vi "initialization.vi"(9 "软件版本":refnum<vi>, 10 "updateconfiguration":refnum<vi>) -> ()   [LabVIEW 2016, in "数据传输系统-02.lvlib"]
uses:
  <vilib>/Utility/config.llb/Read Key (String).vi
  <vilib>/Utility/config.llb/NI_LVConfig.lvlib
  update/update.lvlib
panel:
  in  "参数数值":T1={"CODMn"=TRUE, "CODCr"=TRUE, "DO"=TRUE, "铜"=TRUE, "PH"=TRUE, "氨氮"=TRUE, "比电导率"=TRUE, "水温"=TRUE, "COD"=TRUE, "浊度"=TRUE, "总氮"=TRUE, "总磷"=TRUE, "叶绿素a"=TRUE, "藻密度"=TRUE, "水位"=TRUE, "流速"=TRUE, "瞬时流量"=TRUE, "累积流量"=TRUE, "亚硝氮"=TRUE, "硫化物"=TRUE, "ORP"=TRUE, "铅"=TRUE, "镉"=TRUE, "锌"=TRUE, "镍"=TRUE, "锰"=TRUE, "汞"=TRUE, "气温"=TRUE, "气压"=TRUE, "风速"=TRUE, "风向"=TRUE, "盐度"=TRUE, "磷酸盐"=TRUE, "硝氮"=TRUE, "氟化物"=TRUE}
  out "配置表格":string[][](table)
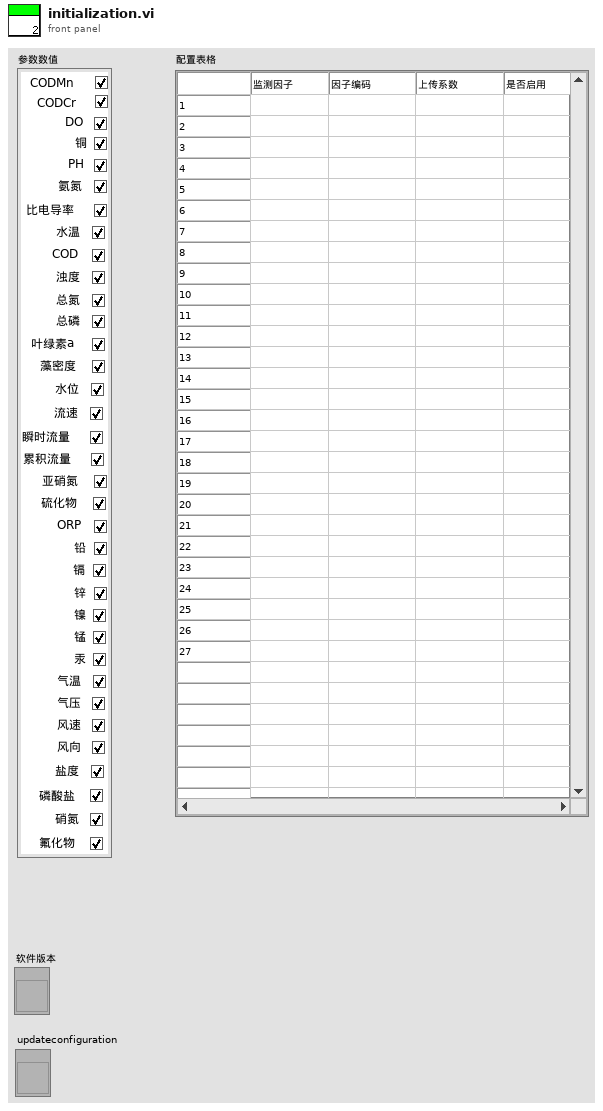
[diagram p1: front panel]
types:
  T1 = cluster{"CODMn":bool, "CODCr":bool, "DO":bool, "铜":bool, "PH":bool, "氨氮":bool, "比电导率":bool, "水温":bool, "COD":bool, "浊度":bool, "总氮":bool, "总磷":bool, "叶绿素a":bool, "藻密度":bool, "水位":bool, "流速":bool, "瞬时流量":bool, "累积流量":bool, "亚硝氮":bool, "硫化物":bool, "ORP":bool, "铅":bool, "镉":bool, "锌":bool, "镍":bool, "锰":bool, "汞":bool, "气温":bool, "气压":bool, "风速":bool, "风向":bool, "盐度":bool, "磷酸盐":bool, "硝氮":bool, "氟化物":bool}
  T2 = cluster{"setini":string, "sysini":string, "hechaini":string, "actualwrite":string, "actualread":string, "datasent":string, "反控命令信息队列":string, "反控与仪器交互":string}
  T3 = cluster{"CODMn":string, "CODCr":string, "DO":string, "铜":string, "PH":string, "氨氮":string, "比电导率":string, "水温":string, "COD":string, "浊度":string, "总氮":string, "总磷":string, "叶绿素a":string, "藻密度":string, "水位":string, "流速":string, "瞬时流量":string, "累积流量":string, "亚硝酸盐":string, "硫化物":string, "ORP":string, "铅":string, "镉":string, "锌":string, "镍":string, "锰":string, "汞":string, "气温":string, "气压":string, "风速":string, "风向":string, "盐度":string, "磷酸盐":string, "硝氮":string, "氟化物":string}
  T4 = typedef "NI_LVConfig.lvlib/Config Data RefNum.ctl" = refnum<k1>
  T5 = cluster{"[0]":string, "[1]":string, "[2]":string, "[3]":string, "[4]":string, "[5]":string, "[6]":string, "[7]":string, "[8]":string, "[9]":string, "[10]":string, "[11]":string, "[12]":string, "[13]":string, "[14]":string, "[15]":string, "[16]":string, "[17]":string, "[18]":string, "[19]":string, "[20]":string, "[21]":string, "[22]":string, "[23]":string, "[24]":string, "[25]":string, "[26]":string, "[27]":string, "[28]":string, "[29]":string, "[30]":string, "[31]":string, "[32]":string, "[33]":string, "[34]":string}
  T6 = cluster{"主机":string, "用户":string, "密码":string, "远程路径":string, "下载文件名":string, "软件版本":string}
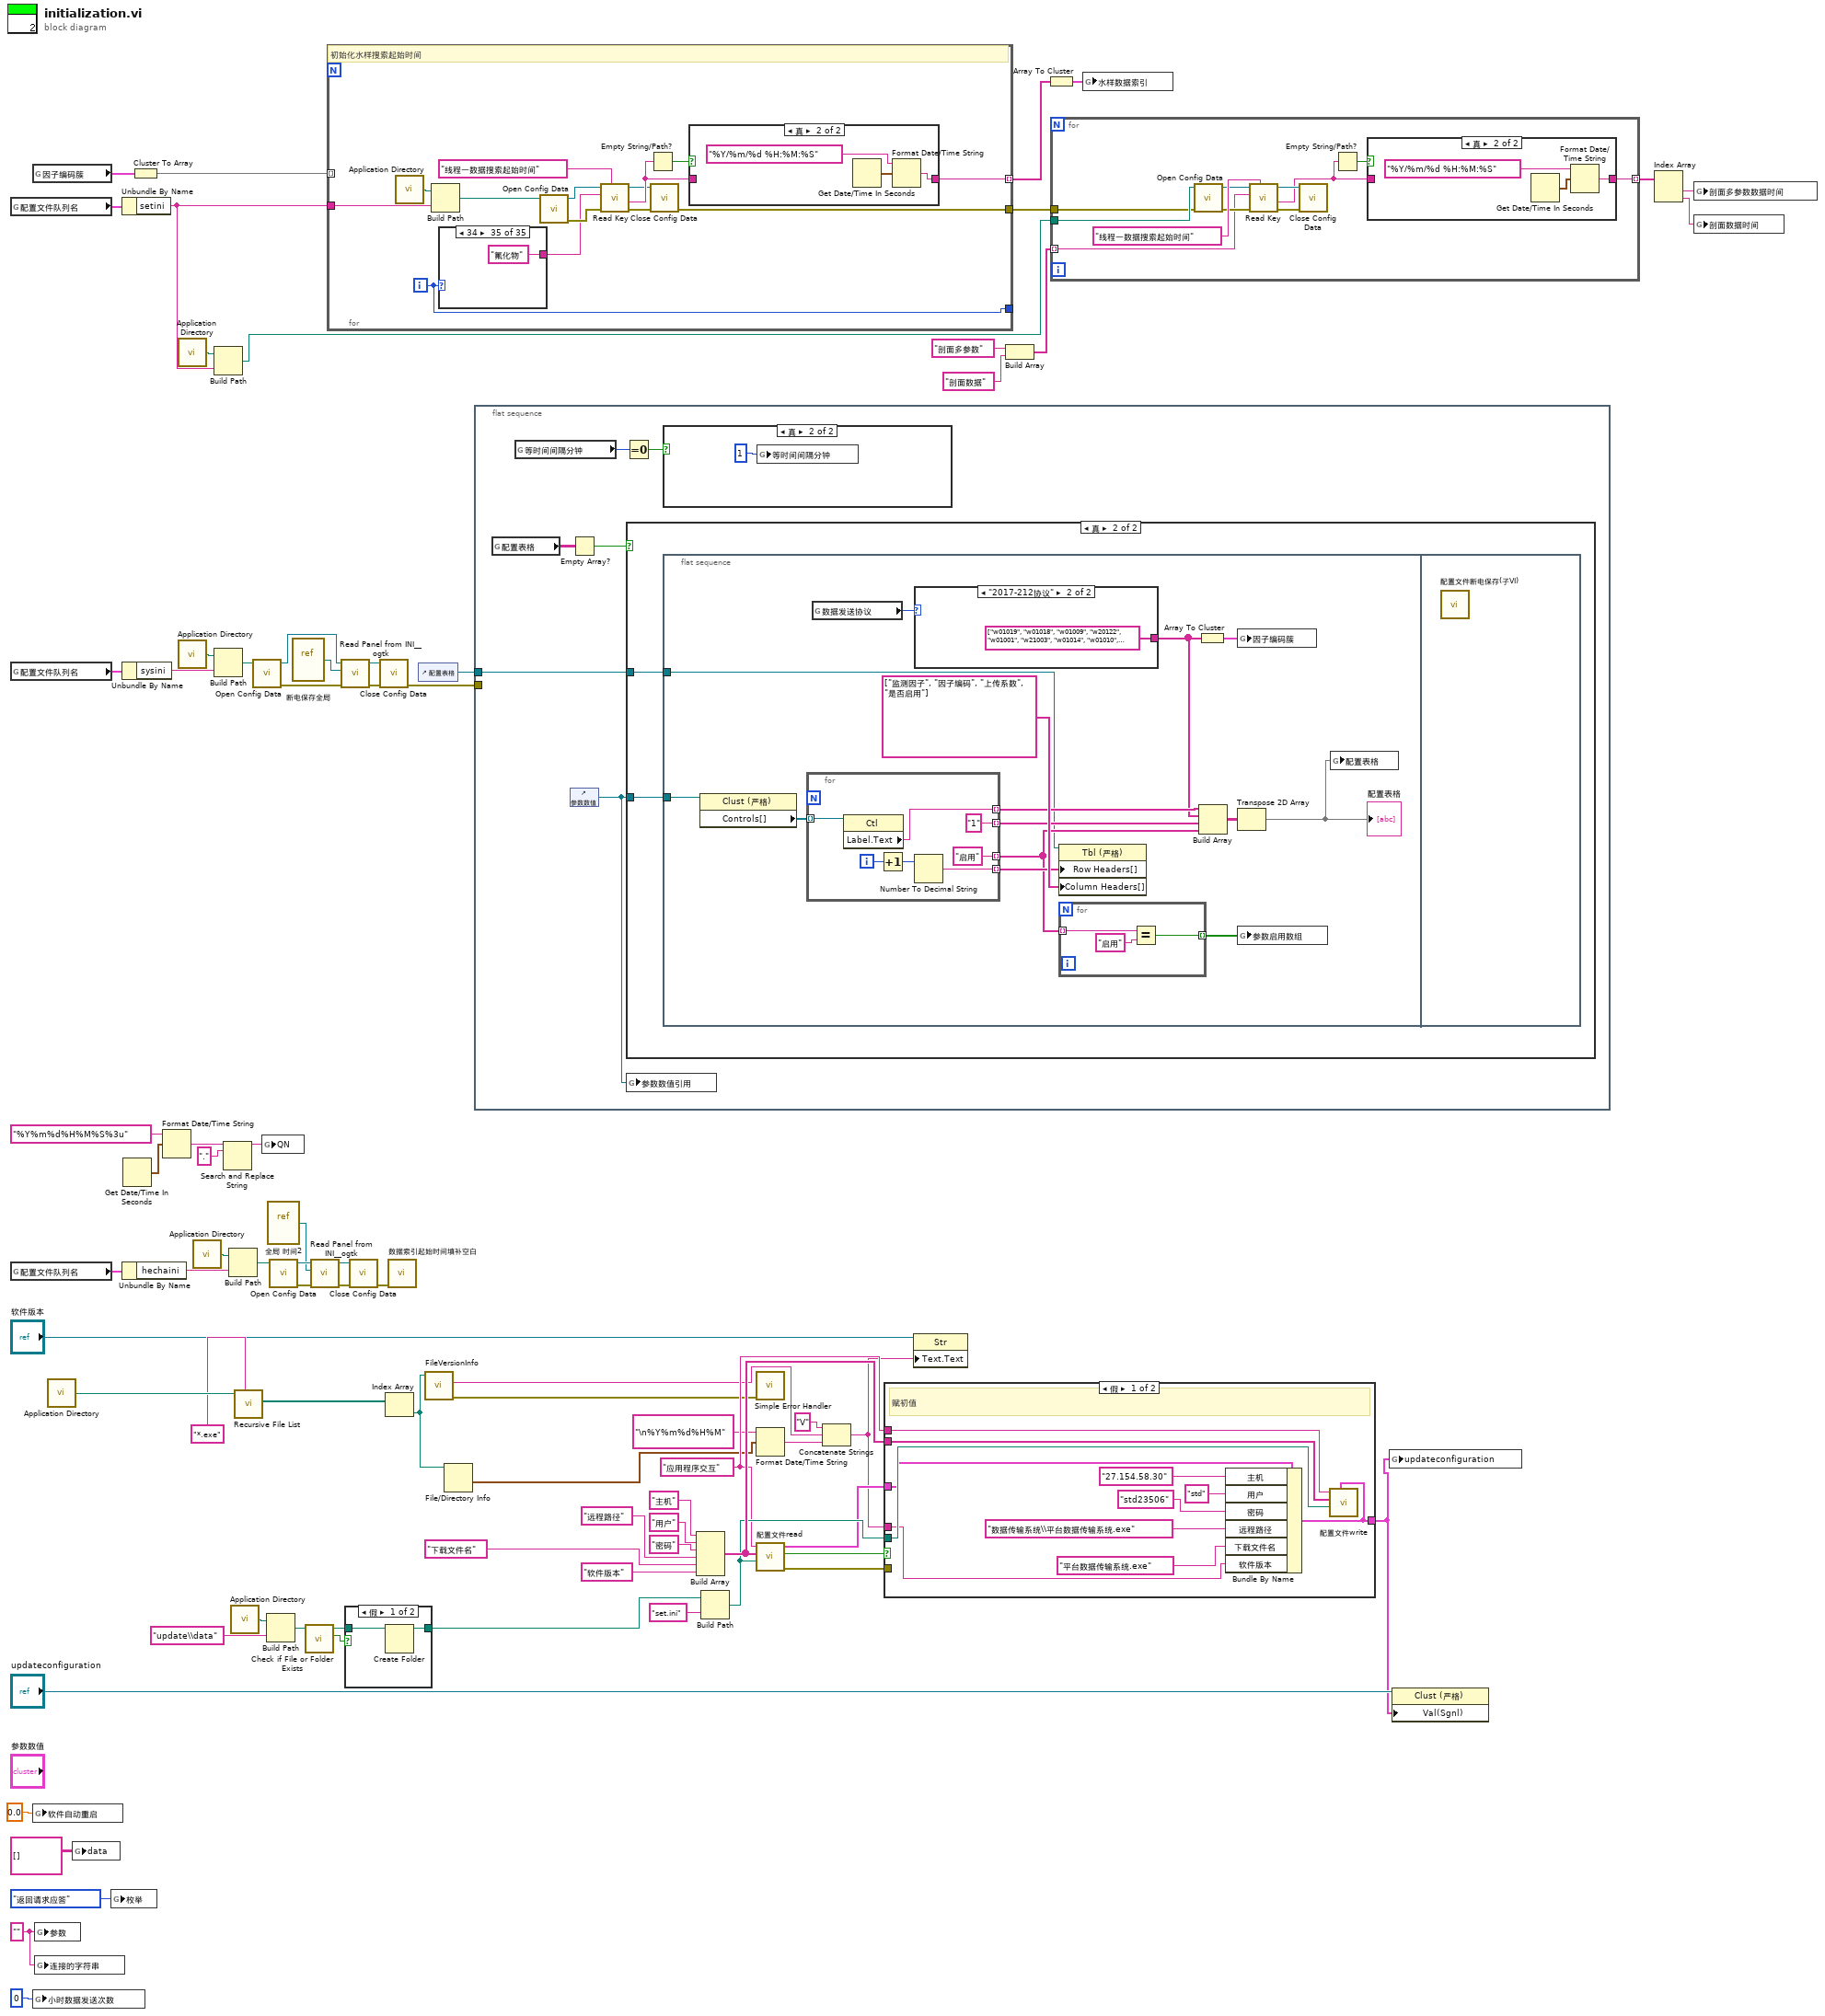
[diagram p0: block diagram]
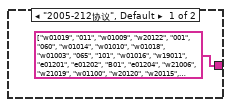
[diagram p4: hidden frame]
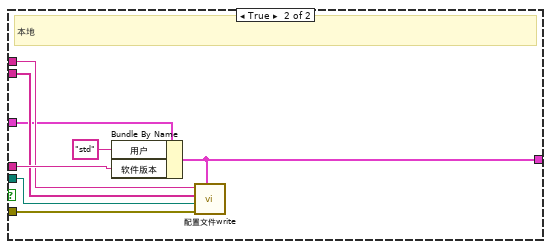
[diagram p7: hidden frame]
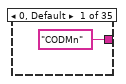
[diagram p9: hidden frame]
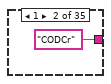
[diagram p10: hidden frame]
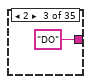
[diagram p11: hidden frame]
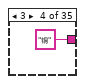
[diagram p12: hidden frame]
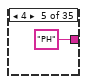
[diagram p13: hidden frame]
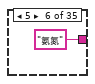
[diagram p14: hidden frame]
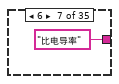
[diagram p15: hidden frame]
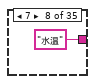
[diagram p16: hidden frame]
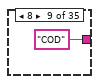
[diagram p17: hidden frame]
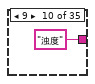
[diagram p18: hidden frame]
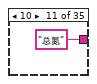
[diagram p19: hidden frame]
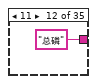
[diagram p20: hidden frame]
diagram:
  w46 = "应用程序交互" ("section")
  w7 = "" ("参数")
  n1 = global read "断电保存全局.vi" "配置文件队列名"() -> (w68:T2)
  n2 = global read "断电保存全局.vi" "配置文件队列名"() -> (w70:T2)
  n3 = global read "断电保存全局.vi" "配置文件队列名"() -> (w72:T2)
  n4 = global read "断电保存全局.vi" "因子编码簇"() -> (w66:T3)
  n5 = global write "全局1.vi" "软件自动重启"(0.0 ("软件自动重启")) -> ()
  n6 = global write "全局 小时数据发送次数.vi" "小时数据发送次数"(0 ("数值")) -> ()
  n7 = global write "全局 实时数据参数.vi" "参数"(w7) -> ()
  n8 = global write "全局 实时数据参数.vi" "连接的字符串"(w7) -> ()
  n9 = call <vilib>:"Application Directory.vi"() -> ("Application Directory"=w22:path)
  n10 = global write "全局 实时数据参数.vi" "data"(string[][] [] ("data")) -> ()
  n11 = global write "全局1.vi" "枚举"(enum16{"返回请求应答", "上传数据", "返回执行结果"}."返回请求应答" ("枚举")) -> ()
  n12 = Unbundle By Name(w68) -> ("setini"=w69:string)
  n13 = Unbundle By Name(w70) -> ("sysini"=w71:string)
  n14 = Unbundle By Name(w72) -> ("hechaini"=w73:string)
  n15 = Get Date/Time In Seconds() -> (seconds since 1Jan1904=w11:timestamp)
  n16 = Cluster To Array(cluster=w66) -> (array=w41:string[])
  n17 = Format Date/Time String(time format string (%c)="%Y%m%d%H%M%S%3u" ("时间格式字符串(%c)"), seconds (now)=w11) -> (date/time string=w12:string)  [unwired: 1 in]
  n18 = call <vilib>:"Application Directory.vi"() -> ("Application Directory"=w62:path)
  n19 = call <vilib>:"Application Directory.vi"() -> ("Application Directory"=w28:path)
  n20 = call <vilib>:"Application Directory.vi"() -> ("Application Directory"=w34:path)
  n21 = Build Path(base path=w62, name or relative path=w69) -> (appended path=w63:path)
  n22 = Build Path(base path=w28, name or relative path=w71) -> (appended path=w29:path)
  n23 = Search and Replace String(input string=w12, search string="." ("搜索字符串")) -> (result string=w14:string)  [unwired: 6 in, 3 out]
  n24 = Build Path(base path=w34, name or relative path=w73) -> (appended path=w33:path)
  n25 = call <vilib>:"Application Directory.vi"() -> ("Application Directory"=w59:path)
  n26 = call <vilib>:"Recursive File List.vi"("pattern"="*.exe", "Folder Path"=w22) -> ("All Files in Dir"=w16:path[])  [unwired: 5 in, 4 out]
  n27 = call <vilib>:"Open Config Data.vi"("configuration file path"=w29) -> ("error out"=w24:errorcluster, "refnum"=w25:T4)  [unwired: 8 in, 1 out]
  n28 = global write "全局1.vi" "QN"(w14) -> ()
  n29 = Build Path(base path=w59, name or relative path="update\\data" ("名称或相对路径")) -> (appended path=w58:path)
  n30 = vi-ref "全局 时间2.vi"() -> (w36:refnum<vi>)
  n31 = call <vilib>:"Open Config Data.vi"("configuration file path"=w33) -> ("error out"=w38:errorcluster, "refnum"=w37:T4)  [unwired: 8 in, 1 out]
  n32 = vi-ref "断电保存全局.vi"() -> (w26:refnum<vi>)
  n33 = call <vilib>:"Check if File or Folder Exists.vi"("path"=w58) -> ("file or folder exists?"=w57:bool, "dup path"=w56:path)  [unwired: 8 in, 1 out]
  n34 = call <userlib>:"Read Panel from INI__ogtk.vi"("error in (no error)"=w38, "VI ref"=w36, "refnum"=w37) -> ("error out"=w39:errorcluster, "refnum out"=w35:T4)  [unwired: 7 in]
  n35 = for {
    tunnel: w41 -> [_] mode=indexing
    tunnel: [w85] -> _
    tunnel: [w82] -> w42 mode=indexing
    tunnel: [w81] -> w64
    tunnel: w69 -> [w80]
    i -> [w85]
    # "初始化水样搜索起始时间"
    n36 = call <vilib>:"Application Directory.vi"() -> ("Application Directory"=w93:path)
    n37 = Build Path(base path=w93, name or relative path=w80) -> (appended path=w92:path)
    n38 = case shown="34" w85 {
      tunnel: ["CODMn" "CODCr" "DO" "铜" "PH" "氨氮" "比电导率" "水温" "COD" "浊度" "总氮" "总磷" "叶绿素a" "藻密度" "水位" "流速" "瞬时流量" "累积流量" "亚硝氮" "硫化物" "ORP" "铅" "镉" "锌" "镍" "锰" "汞" "气温" "气压" "风速" "风向" "盐度" "磷酸盐" "硝氮" "氟化物"] -> w88
      frame 0, Default {
      }
      frame 1 {
      }
      frame 2 {
      }
      frame 3 {
      }
      frame 4 {
      }
      frame 5 {
      }
      frame 6 {
      }
      frame 7 {
      }
      frame 8 {
      }
      frame 9 {
      }
      frame 10 {
      }
      frame 11 {
      }
      frame 12 {
      }
      frame 13 {
      }
      frame 14 {
      }
      frame 15 {
      }
      frame 16 {
      }
      frame 17 {
      }
      frame 18 {
      }
      frame 19 {
      }
      frame 20 {
      }
      frame 21 {
      }
      frame 22 {
      }
      frame 23 {
      }
      frame 24 {
      }
      frame 25 {
      }
      frame 26 {
      }
      frame 27 {
      }
      frame 28 {
      }
      frame 29 {
      }
      frame 30 {
      }
      frame 31 {
      }
      frame 32 {
      }
      frame 33 {
      }
      frame 34 {
      }
    }
    n39 = call <vilib>:"Open Config Data.vi"("configuration file path"=w92) -> ("error out"=w90:errorcluster, "refnum"=w91:T4)  [unwired: 8 in, 1 out]
    n40 = call-poly <vilib>:"Read Key.vi"("section"="线程一数据搜索起始时间", "error in (no error)"=w90, "key"=w88, "refnum"=w91) -> ("error out"=w83:errorcluster, "value"=w86:string, "refnum out"=w84:T4)  [unwired: 4 in, 1 out]
    n41 = Empty String/Path?(string/path=w86) -> (empty?=w87:bool)
    n42 = call <vilib>:"Close Config Data.vi"("error in (no error)"=w83, "refnum"=w84) -> ("error out"=w81:errorcluster)  [unwired: 8 in, 1 out]
    n43 = case shown="真" w87 {
      tunnel: [w94 w95] -> w82
      tunnel: w86 -> [w94 _]
      frame False {
      }
      frame True {
        n44 = Get Date/Time In Seconds() -> (seconds since 1Jan1904=w97:timestamp)
        n45 = Format Date/Time String(time format string (%c)="%Y/%m/%d %H:%M:%S" ("时间格式字符串(%c)"), seconds (now)=w97) -> (date/time string=w95:string)  [unwired: 1 in]
      }
    }
  }
  n46 = call <userlib>:"Read Panel from INI__ogtk.vi"("error in (no error)"=w24, "VI ref"=w26, "refnum"=w25) -> ("error out"=w30:errorcluster, "refnum out"=w27:T4)  [unwired: 7 in]
  n47 = case shown="假" w57 {
    tunnel: w56 -> [w134 w135]
    tunnel: [w133 w135] -> w61
    frame False {
      n48 = Create Folder(path (use dialog)=w134) -> (created path=w133:path)  [unwired: 2 in, 2 out]
    }
    frame True {
    }
  }
  n49 = call <vilib>:"Close Config Data.vi"("error in (no error)"=w39, "refnum"=w35) -> ("error out"=w40:errorcluster)  [unwired: 8 in, 1 out]
  n50 = call <vilib>:"Close Config Data.vi"("error in (no error)"=w30, "refnum"=w27) -> ("error out"=w65:errorcluster)  [unwired: 8 in, 1 out]
  n51 = Index Array(array=w16) -> (element=w17:path)  [unwired: 1 in]
  n52 = call "数据索引起始时间填补空白.vi"("error in (no error)"=w40) -> ()  [unwired: 10 in, 1 out]
  n53 = control-ref of="配置表格"() -> (w4:refnum<vi>)
  n54 = call <vilib>:"FileVersionInfo.vi"("Application Path in"=w17) -> ("error out"=w23:errorcluster, "File Version Info"=w32:string)  [unwired: 7 in, 2 out]
  n55 = File/Directory Info(path=w17) -> (last mod=w18:timestamp)  [unwired: 1 in, 6 out]
  n56 = flat-sequence {
    tunnel: w65 -> [_]
    tunnel: w4 -> [w139]
    frame #0 {
      n57 = global read "断电保存全局.vi" "配置表格"() -> (w141:string[][])
      n58 = global read "断电保存全局.vi" "等时间间隔分钟"() -> (w136:i32)
      n59 = Empty Array?(array=w141) -> (empty?=w140:bool)
      n60 = control-ref of="参数数值"() -> (w138:refnum<vi>)
      n61 = Equal To 0?(x=w136) -> (x = 0?=w137:bool)
      n62 = case shown="真" w140 {
        tunnel: w139 -> [_ w144]
        tunnel: w138 -> [_ w143]
        frame False {
        }
        frame True {
          n63 = flat-sequence {
            tunnel: w144 -> [w146]
            tunnel: w143 -> [w145]
            frame #0 {
              n64 = property on="属性节点" class="Clust (严格)"(reference=w145) -> ("Controls[]"=w154:refnum<vi>[])  [unwired: 1 in, 2 out]
              n65 = for {
                tunnel: w154 -> [w170] mode=indexing
                tunnel: [w169] -> w156 mode=indexing
                tunnel: [w167] -> w155 mode=indexing
                tunnel: ["1"] -> w149 mode=indexing
                tunnel: ["启用"] -> w148 mode=indexing
                i -> [w168]
                n66 = property class="Ctl"(reference=w170) -> ("Label.Text"=w169:string)  [unwired: 1 in, 2 out]
                n67 = Increment(x=w168) -> (x+1=w166:i32)
                n68 = Number To Decimal String(number=w166) -> (decimal integer string=w167:string)  [unwired: 1 in]
              }
              n69 = global read "断电保存全局.vi" "数据发送协议"() -> (w152:enum16{"2005-212协议", "2017-212协议"})
              n70 = case shown="\"2017-212协议\"" w152 {
                tunnel: [string[] ["w01019", "011", "w01009", "w20122", "001", "060", "w01014", "w01010", "w01018", "w01003", "065", "101", "w01016", "w19011", "e01201", "e01202", "B01", "e01204", "w21006", "w21019", "w01100", "w20120", "w20115", "w20123", "w20121", "w20124", "w20111", "a01001", "a01006", "a01007", "a01008", "w01002", "w21015", "w21007", "w21017"] string[] ["w01019", "w01018", "w01009", "w20122", "w01001", "w21003", "w01014", "w01010", "w01018", "w01003", "w21001", "w21011", "w01016", "w19011", "e01201", "e01202", "e01203", "e01204", "w21006", "w21019", "w01100", "w20120", "w20115", "w20123", "w20121", "w20124", "w20111", "a01001", "a01006", "a01007", "a01008", "w01002", "w21015", "w21007", "w21017"]] -> w150
                frame "2005-212协议", Default {
                }
                frame "2017-212协议" {
                }
              }
              n71 = property on="属性节点" class="Tbl (严格)"(reference=w146, "Row Headers[]"=w155, "Column Headers[]"=string[] ["监测因子", "因子编码", "上传系数", "是否启用"]) -> ()  [unwired: 1 in, 2 out]
              n72 = for {
                tunnel: w148 -> [w161] mode=indexing
                tunnel: [w159] -> w147 mode=indexing
                n73 = Equal?(x=w161, y="启用") -> (x = y?=w159:bool)
              }
              n74 = Array To Cluster(array=w150) -> (cluster=w151:T5)
              n75 = Build Array(w156, w150, w149, w148) -> (w158:string[][])
              n76 = global write "断电保存全局.vi" "因子编码簇"(w151) -> ()
              n77 = Transpose 2D Array(2D array=w158) -> (transposed array=w153:string[][])
              "配置表格" <- w153
              n78 = global write "断电保存全局.vi" "参数启用数组"(w147) -> ()
              n79 = global write "断电保存全局.vi" "配置表格"(w153) -> ()
            }
            frame #1 {
              n80 = call "配置文件断电保存(子VI).vi"() -> ()  [unwired: 12 in]
            }
          }
        }
      }
      n81 = global write "断电保存全局.vi" "参数数值引用"(w138) -> ()
      n82 = case shown="真" w137 {
        frame False {
        }
        frame True {
          n83 = global write "断电保存全局.vi" "等时间间隔分钟"(1 ("等时间间隔分钟")) -> ()
        }
      }
    }
  }
  n84 = Build Array("主机" ("section"), "用户" ("section"), "密码" ("key"), "远程路径" ("key"), "下载文件名" ("key"), "软件版本" ("key")) -> (w55:string[])
  n85 = Build Path(base path=w61, name or relative path="set.ini" ("名称或相对路径")) -> (appended path=w47:path)
  n86 = call <vilib>:"Simple Error Handler.vi"("error in (no error)"=w23) -> ()  [unwired: 4 in, 5 out]
  n87 = Format Date/Time String(time format string (%c)="\n%Y%m%d%H%M" ("时间格式字符串(%c)"), seconds (now)=w18) -> (date/time string=w21:string)  [unwired: 1 in]
  n88 = call "配置文件read.vi"("configuration file path"=w47, "键数组"=w55, "段"=w46) -> ("error out"=w48:errorcluster, "section exists?"=w44:bool, "updateconfiguration"=w45:T6)  [unwired: 6 in]
  n89 = Concatenate Strings("V" ("字符串"), w32, w21) -> (w2:string)
  n90 = case shown="假" w44 {
    tunnel: w45 -> [w177 w184]
    tunnel: [w176 w183] -> w1
    tunnel: w2 -> [w171 w189]
    tunnel: w46 -> [w180 w188]
    tunnel: w55 -> [w179 w187]
    tunnel: w47 -> [w178 w186]
    tunnel: w48 -> [_ w185]
    frame False {
      # "赋初值"
      n91 = Bundle By Name(cluster=w177, "主机"="27.154.58.30" ("key"), "用户"="std", "密码"="std23506", "远程路径"="数据传输系统\\平台数据传输系统.exe", "下载文件名"="平台数据传输系统.exe", "软件版本"=w171) -> (w176:T6)
      n92 = call "配置文件write.vi"("updateconfiguration"=w176, "configuration file path"=w178, "键数组"=w179, "段"=w180) -> ()  [unwired: 7 in, 1 out]
    }
    frame True {
      # "本地"
      n93 = Bundle By Name(cluster=w184, "用户"="std", "软件版本"=w189) -> (w183:T6)
      n94 = call "配置文件write.vi"("updateconfiguration"=w183, "error in (no error)"=w185, "configuration file path"=w186, "键数组"=w187, "段"=w188) -> ()  [unwired: 6 in, 1 out]
    }
  }
  n95 = property class="Str"(reference="软件版本", "Text.Text"=w2) -> ()  [unwired: 1 in, 2 out]
  n96 = Build Array("剖面多参数" ("key"), "剖面数据" ("key")) -> (w76:string[])
  n97 = Array To Cluster(array=w42) -> (cluster=w43:T5)
  n98 = for {
    tunnel: w63 -> [w200]
    tunnel: w64 -> [w199]
    tunnel: w76 -> [w191] mode=indexing
    tunnel: [w190] -> w77 mode=indexing
    n99 = call <vilib>:"Open Config Data.vi"("error in (no error)"=w199, "configuration file path"=w200) -> ("error out"=w196:errorcluster, "refnum"=w197:T4)  [unwired: 7 in, 1 out]
    n100 = call-poly <vilib>:"Read Key.vi"("section"="线程一数据搜索起始时间", "error in (no error)"=w196, "key"=w191, "refnum"=w197) -> ("error out"=w194:errorcluster, "value"=w193:string, "refnum out"=w195:T4)  [unwired: 4 in, 1 out]
    n101 = call <vilib>:"Close Config Data.vi"("error in (no error)"=w194, "refnum"=w195) -> ()  [unwired: 8 in, 2 out]
    n102 = Empty String/Path?(string/path=w193) -> (empty?=w192:bool)
    n103 = case shown="真" w192 {
      tunnel: [w201 w202] -> w190
      tunnel: w193 -> [w201 _]
      frame False {
      }
      frame True {
        n104 = Get Date/Time In Seconds() -> (seconds since 1Jan1904=w204:timestamp)
        n105 = Format Date/Time String(time format string (%c)="%Y/%m/%d %H:%M:%S" ("时间格式字符串(%c)"), seconds (now)=w204) -> (date/time string=w202:string)  [unwired: 1 in]
      }
    }
  }
  n106 = global write "全局 水样时间.vi" "水样数据索引"(w43) -> ()
  n107 = global write "更新全局变量.vi" "updateconfiguration"(w1) -> ()
  n108 = property on="属性节点" class="Clust (严格)"(reference="updateconfiguration", "Val(Sgnl)"=w1) -> ()  [unwired: 1 in, 2 out]
  n109 = Index Array(array=w77) -> (element #1=w78:string, element #2=w79:string)  [unwired: 2 in]
  n110 = global write "全局 水样时间.vi" "剖面多参数数据时间"(w78) -> ()
  n111 = global write "全局 水样时间.vi" "剖面数据时间"(w79) -> ()
